vi "Read Attributes.vi"(11 "NS Connection Msg":refnum<class "NS Connection Msg.lvclass">) -> (2 "Payload":cluster{"NS Conn":bool})   [LabVIEW 2019, in "Network Stream.lvlib" / "NS Connection Msg.lvclass"]
uses:
  NS Connection Msg.lvclass
  NS Connection Msg.lvclass/NS Connection Msg.ctl
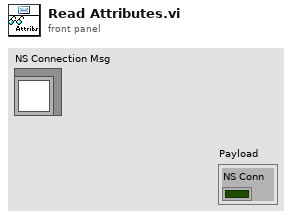
[diagram p1: front panel]
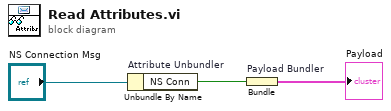
[diagram p0: block diagram]
diagram:
  n1 = Unbundle By Name "Attribute Unbundler"("NS Connection Msg") -> ("NS Conn"=w1:bool)
  n2 = Bundle "Payload Bundler"("NS Conn"=w1) -> (→"Payload":cluster{"NS Conn":bool})  [unwired: 1 in]
